vi "PID.vi"(6 "reinitialize? (F)":bool, 8 "error in (no error)":errorcluster) -> (0 "error out":errorcluster, 2 "Y output":dbl(slide) scale=-50.0..50.0, 3 "X output":dbl(slide) scale=-50.0..50.0)   [LabVIEW 2016]
uses:
  <vilib>/addons/control/pid/pid.llb/PID (DBL).vi
  <vilib>/addons/control/pid/NI_PID_pid.lvlib
panel:
  out "Y Servo Angle":i16(slide) scale=0.0..100.0
  out "X Servo Angle":i16(slide) scale=0.0..100.0
  out "Y_PV":dbl
  out "X_PV":dbl
  out "dt out (s)":dbl format="%.3f"
  in  "output range":cluster{"output high":dbl, "output low":dbl}={"output high"=50.0, "output low"=-50.0} {"output low" format="%.2f"; "output high" format="%.2f"}
  in  "dt (s)":dbl=-1.0 format="%.3f"
  in  "PID gains":T1={"proportional gain (Kc)"=1.0, "integral time (Ti, min)"=0.01, "derivative time (Td, min)"=0.0} {"derivative time (Td, min)" format="%.3f"; "integral time (Ti, min)" format="%.3f"; "proportional gain (Kc)" format="%.3f"}
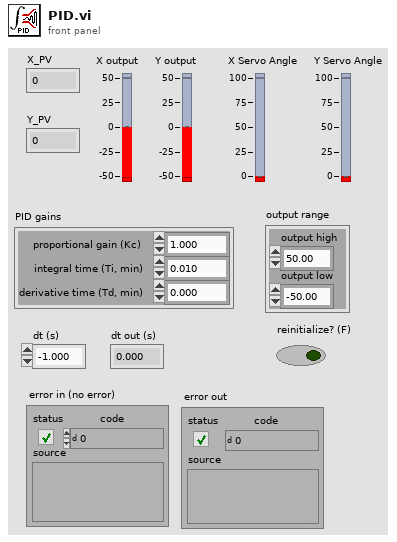
[diagram p1: front panel]
types:
  T1 = cluster{"proportional gain (Kc)":dbl, "integral time (Ti, min)":dbl, "derivative time (Td, min)":dbl}
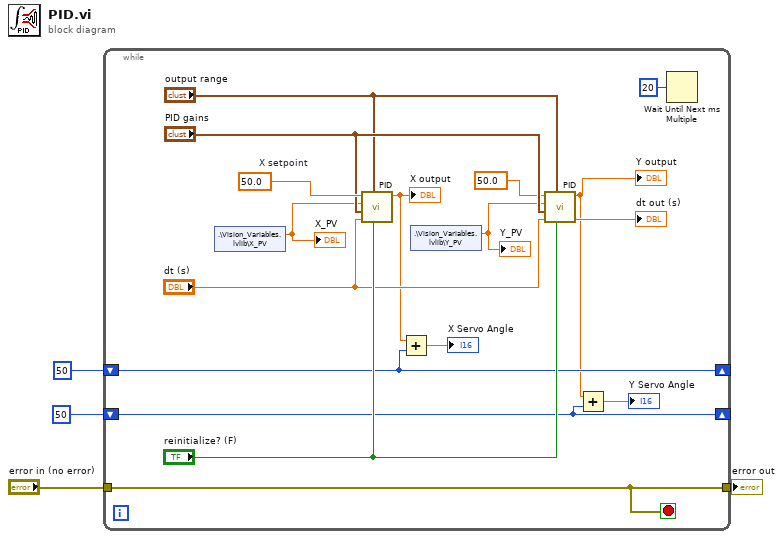
[diagram p0: block diagram]
diagram:
  n1 = while {
    tunnel: [w13] -> w4
    tunnel: "error in (no error)" -> [w13]
    shift-right: [w5] -> _
    shift-left: 50 -> [w5]
    shift-right: [w8] -> _
    shift-left: 50 -> [w8]
    stop <- w13 stop-if-true
    w21 = 50.0  # X setpoint
    n2 = shared-variable ".\\Vision_Variables.lvlib\\X_PV"() -> (w12:dbl)  [unwired: 1 in, 1 out]
    "X_PV" <- w12
    n3 = call-poly <vilib>:"PID.vi"("reinitialize? (F)"="reinitialize? (F)", "output range"="output range", "dt (s)"="dt (s)", "PID gains"="PID gains", "process variable"=w12, "setpoint"=w21) -> ("output"=w9:dbl)  [unwired: 4 in, 1 out]
    "X output" <- w9
    n4 = Add(x=w9, y=w8) -> (x+y=→"X Servo Angle":dbl)
    n5 = shared-variable ".\\Vision_Variables.lvlib\\Y_PV"() -> (w11:dbl)  [unwired: 1 in, 1 out]
    "Y_PV" <- w11
    n6 = call-poly <vilib>:"PID.vi"("reinitialize? (F)"="reinitialize? (F)", "output range"="output range", "dt (s)"="dt (s)", "PID gains"="PID gains", "process variable"=w11, "setpoint"=50.0 ("Y setpoint")) -> ("dt out (s)"=→"dt out (s)":dbl, "output"=w6:dbl)  [unwired: 4 in]
    "Y output" <- w6
    n7 = Add(x=w6, y=w5) -> (x+y=→"Y Servo Angle":dbl)
    n8 = Wait Until Next ms Multiple(millisecond multiple=u32 20) -> ()  [unwired: 1 out]
  }
  "error out" <- w4
